vi "ConvertingC_2_F.vi"() -> ()   [LabVIEW 2015]
panel:
  in  "Boolean":bool
  in  "stop":bool
  out "Degrees F":dbl(slide) scale=0.0..300.0
  in  "Degrees C":dbl(slide) scale=0.0..150.0
  # "INPUT DEGREES C"
  # "OUTPUT IN DEGREES F"
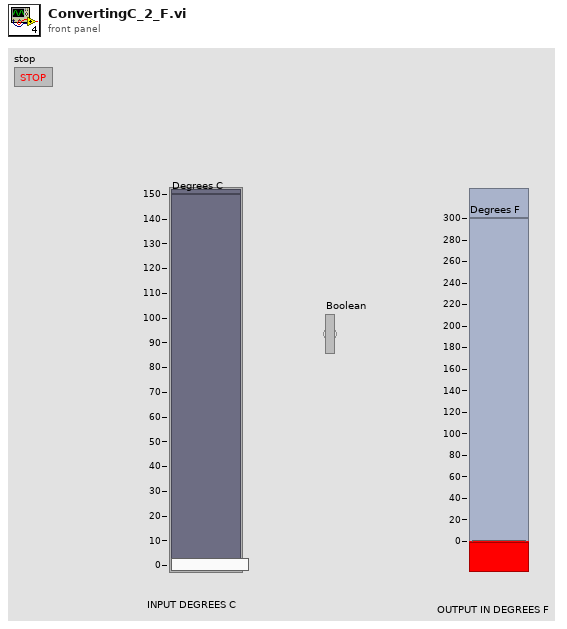
[diagram p1: front panel]
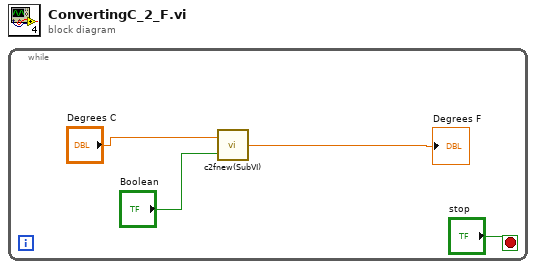
[diagram p0: block diagram]
diagram:
  n1 = while {
    stop <- "stop" stop-if-true
    n2 = call "c2fnew(SubVI).vi"("Boolean"="Boolean", "Degrees C"="Degrees C") -> ("Numeric"=→"Degrees F":dbl)
  }
